vi "example_dll.vi"(8 "Error In":errorcluster) -> (0 "Error Out":errorcluster)   [LabVIEW 2014]
panel:
  out "number out":i32
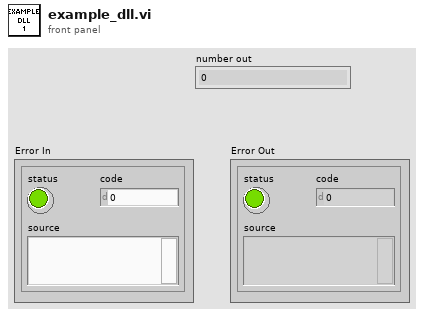
[diagram p1: front panel]
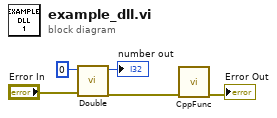
[diagram p0: block diagram]
diagram:
  n1 = call "Double.vi"("Error In"="Error In", "number in"=0) -> ("Error Out"=w1:errorcluster, "number out"=→"number out":i32)  [unwired: 8 in]
  n2 = call "CppFunc.vi"("Error In"=w1) -> ("Error Out"=→"Error Out":errorcluster)  [unwired: 10 in]
